vi "PositionBased1DProfile.vi"(9 "MaxAccel":dbl, 10 "MaxVel":dbl, 11 "Distance":dbl) -> (3 "Profile":cluster{"Distances":dbl[], "Vels":dbl[]})   [LabVIEW 2017]
panel:
  out "XY Graph":cluster{dbl[], dbl[]}(graph)
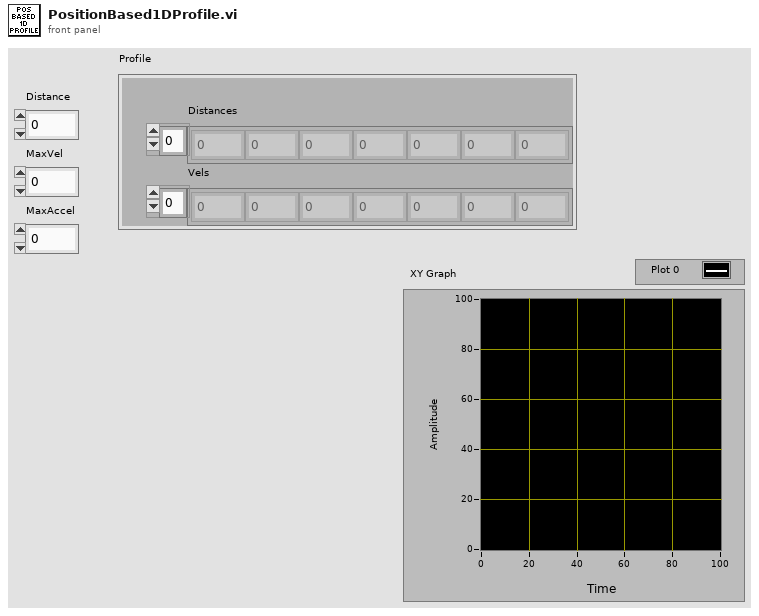
[diagram p1: front panel]
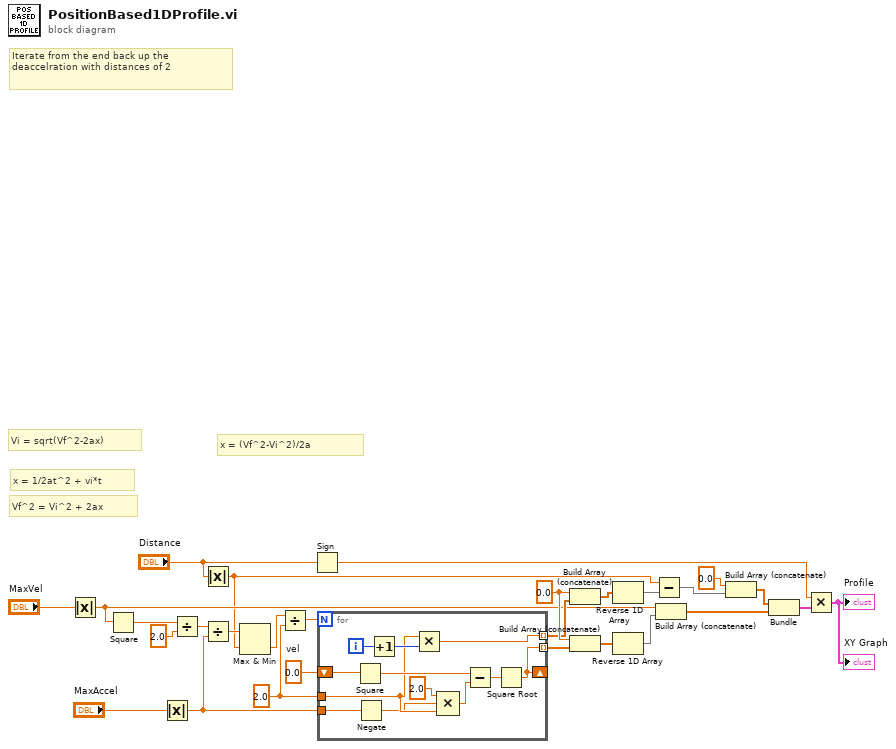
[diagram p0: block diagram]
diagram:
  w18 = 0.0 ("y")
  w24 = 0.0  # vel
  w25 = 2.0 ("y")
  # "Vi = sqrt(Vf^2-2ax)"
  # "Iterate from the end back up the\ndeaccelration with distances of 2"
  # "x = (Vf^2-Vi^2)/2a"
  # "Vf^2 = Vi^2 + 2ax"
  # "x = 1/2at^2 + vi*t"
  n1 = Absolute Value(x="MaxVel") -> (abs(x)=w8:dbl)
  n2 = Square(x=w8) -> (x^2=w26:dbl)
  n3 = Absolute Value(x="MaxAccel") -> (abs(x)=w6:dbl)
  n4 = Divide(x=w26, y=2.0) -> (x/y=w27:dbl)
  n5 = Absolute Value(x="Distance") -> (abs(x)=w5:dbl)
  n6 = Divide(x=w27, y=w6) -> (x/y=w20:dbl)
  n7 = Max & Min(x=w20, y=w5) -> (min(x,y)=w11:dbl)  [unwired: 1 out]
  n8 = Divide(x=w11, y=w25) -> (x/y=w19:dbl)
  n9 = Sign(1:"Distance") -> (0:w2:dbl)
  n10 = for {
    N: w19 -> [_]
    tunnel: w25 -> [w35]
    shift-right: [w32] -> _
    shift-left: w24 -> [w38]
    tunnel: w6 -> [w31]
    tunnel: [w32] -> w17 mode=indexing
    tunnel: [w29] -> w16 mode=indexing
    i -> [w40]
    n11 = Square(x=w38) -> (x^2=w37:dbl)
    n12 = Negate(x=w31) -> (-x=w30:dbl)
    n13 = Increment(x=w40) -> (x+1=w39:i32)
    n14 = Multiply(x=w35, y=w39) -> (x*y=w29:dbl)
    n15 = Compound Arithmetic op=MULTIPLY(2.0 ("value"), w30, w35) -> (w34:dbl)
    n16 = Subtract(x=w37, y=w34) -> (x-y=w33:dbl)
    n17 = Square Root(x=w33) -> (sqrt(x)=w32:dbl)
  }
  n18 = Build Array (concatenate)(w18, w16) -> (w15:dbl[])
  n19 = Build Array (concatenate)(w18, w17) -> (w23:dbl[])
  n20 = Reverse 1D Array(array=w15) -> (reversed array=w12:dbl[])
  n21 = Reverse 1D Array(array=w23) -> (reversed array=w13:dbl[])
  n22 = Subtract(x=w5, y=w12) -> (x-y=w10:dbl[])
  n23 = Build Array (concatenate)(w8, w13) -> (w21:dbl[])
  n24 = Build Array (concatenate)(0.0 ("y"), w10) -> (w22:dbl[])
  n25 = Bundle(w22, w21) -> (w3:cluster{dbl[], dbl[]})  [unwired: 1 in]
  n26 = Multiply(x=w2, y=w3) -> (x*y=→"Profile" →"XY Graph":cluster{dbl[], dbl[]})
